vi "Create file.vi"(8 "error in (no error)":errorcluster, 9 "Parent":refnum<class "system object.lvclass">, 10 "size":i32, 11 "name":string) -> (0 "error out":errorcluster, 3 "File out":refnum<class "File.lvclass">)   [LabVIEW 2020, in "File.lvclass"]
uses:
  File.lvclass
  C:/PA_Source/advent-of-code/2022/Paul/07/classes/system object/system object.lvclass
  system object/system object.lvclass
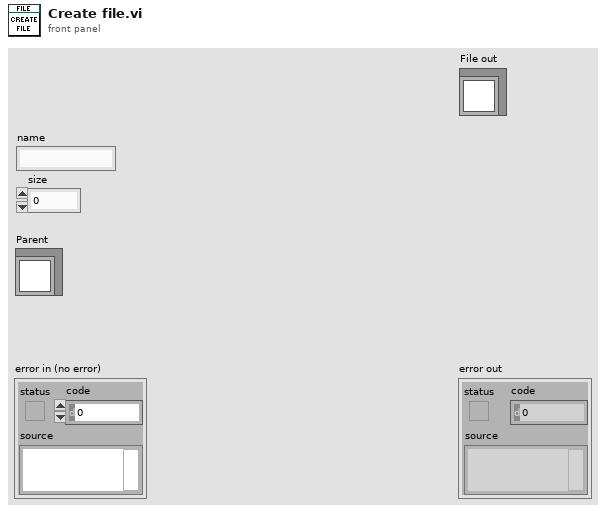
[diagram p1: front panel]
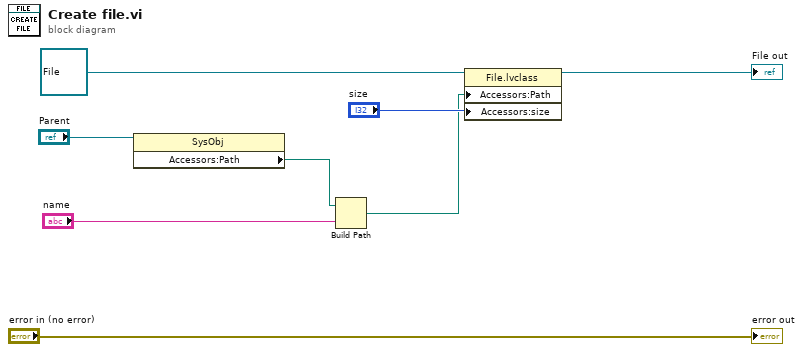
[diagram p0: block diagram]
diagram:
  n1 = property class="SysObj"(reference="Parent") -> ("Accessors:Path"=w3:path)  [unwired: 1 in, 2 out]
  n2 = Build Path(base path=w3, name or relative path="name") -> (appended path=w1:path)
  n3 = property class="File.lvclass"(reference=refnum<class "File.lvclass"> refnum ("File in"), "Accessors:Path"=w1, "Accessors:size"="size") -> (reference out=→"File out":refnum<class "File.lvclass">)  [unwired: 1 in, 1 out]
  "error out" <- "error in (no error)"
